vi "不同波形频率声卡输出.vi"() -> ()   [LabVIEW 2019]
uses:
  <vilib>/measure/NI_MABase.lvlib
panel:
  in  "停止":bool
  out "波形图":waveform(dbl)(graph)
  in  "下拉列表":u16(ring) items=["正弦波", "三角波", "方波", "锯齿波"]
  in  "方波占空比":dbl format="%#_13g"
  in  "采样点数":dbl format="%#_13g"
  in  "采样频率":dbl format="%#_13g"
  in  "信号频率":dbl format="%#_13g"
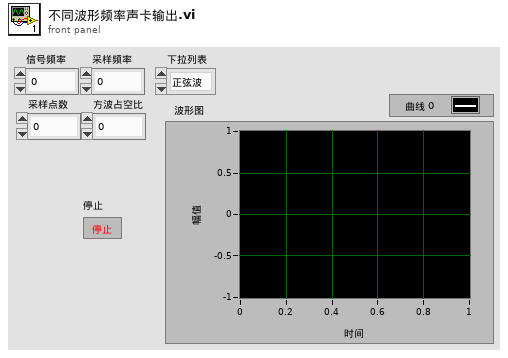
[diagram p1: front panel]
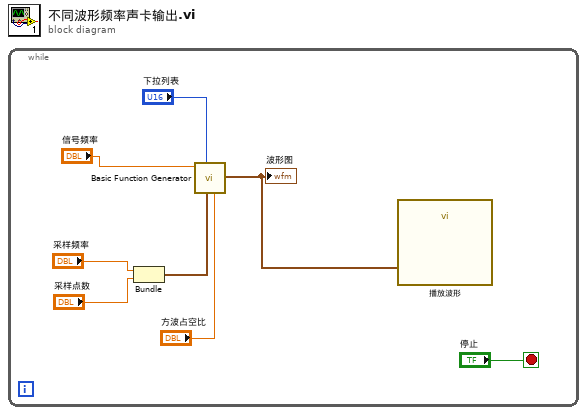
[diagram p0: block diagram]
diagram:
  n1 = while {
    stop <- "停止" stop-if-true
    n2 = Bundle("采样频率"="采样频率", "采样点数"="采样点数") -> (w6:cluster{"采样频率":dbl, "采样点数":dbl})  [unwired: 1 in]
    n3 = call <vilib>:"Basic Function Generator.vi"("square wave duty cycle (%)"="方波占空比", "sampling info"=w6, "signal type"="下拉列表", "frequency"="信号频率") -> ("signal out"=w2:waveform(dbl))  [unwired: 5 in, 2 out]
    "波形图" <- w2
    n4 = call "播放波形"("Data"=w2) -> ()  [unwired: 18 in, 1 out]
  }
